vi "Select DB data(Count).vi"(6 "index":i32, 8 "error in (no error)":errorcluster caption="错误输入（无错误）", 9 "Code":string, 10 "Tabe":string, 11 "Connncet State":T1) -> (0 "error out":errorcluster caption="错误输出", 2 "state":bool, 3 "Connect State":T1)   [LabVIEW 2014]
uses:
  Ctr/Conneect State.ctl
  Ctr/Constr.ctl
  <vilib>/addons/database/Connection.llb/Conn ObjectReference.ctl
  <vilib>/addons/database/NI_Database_API.lvlib
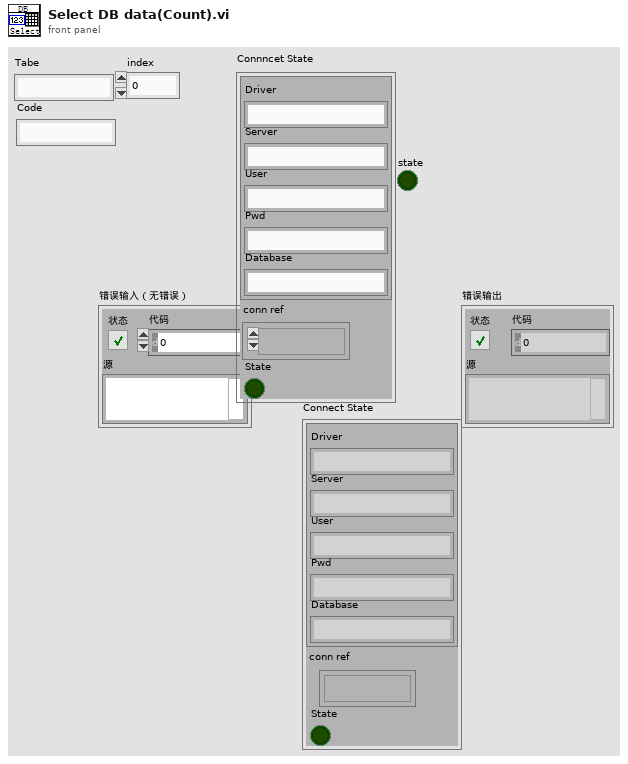
[diagram p1: front panel]
types:
  T1 = typedef "Conneect State.ctl" = cluster{"Constr":T2, "conn ref":T3, "State":bool}
  T2 = typedef "Constr.ctl" = cluster{"Driver":string, "Server":string, "User":string, "Pwd":string, "Database":string}
  T3 = typedef "NI_Database_API.lvlib/Conn ObjectReference.ctl" = refnum<k1>
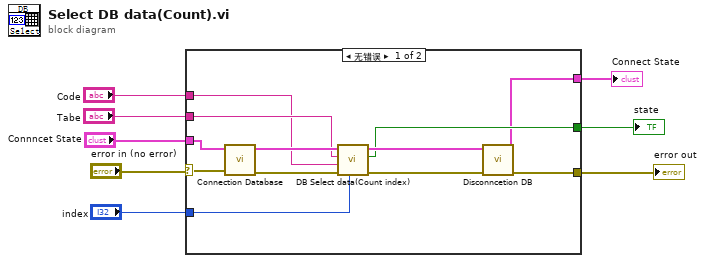
[diagram p0: block diagram]
diagram:
  n1 = case shown="无错误" "error in (no error)" {
    selector: "error in (no error)" -> [w20 w22]
    tunnel: "Connncet State" -> [w19 w21]
    tunnel: [w15 w22] -> w6
    tunnel: "Tabe" -> [w14 _]
    tunnel: "Code" -> [w13 _]
    tunnel: "index" -> [w12 _]
    tunnel: [w11 _] -> w2
    tunnel: [w10 w21] -> w1
    frame No Error {
      n2 = call "Connection Database.vi"("error in (no error)"=w20, "Connncet State"=w19) -> ("error out"=w18:errorcluster, "Connncet State out"=w17:T1)  [unwired: 8 in]
      n3 = call "DB Select data(Count index).vi"("index"=w12, "error in (no error)"=w18, "Code"=w13, "Tabe"=w14, "Connncet State"=w17) -> ("error out"=w9:errorcluster, "state"=w11:bool, "Connncet State out"=w16:T1)  [unwired: 3 in, 1 out]
      n4 = call "Disconncetion DB.vi"("error in (no error)"=w9, "Connncet State"=w16) -> ("error out"=w15:errorcluster, "Connect State"=w10:T1)  [unwired: 8 in]
    }
    frame Error {
    }
  }
  "error out" <- w6
  "state" <- w2
  "Connect State" <- w1
